vi "регистр на RSDC(фронтовой).vi"(2 "C":bool, 3 "S":bool, 4 "R":bool, 5 "d":T3) -> (0 "not q":T1, 1 "q":T2)   [LabVIEW 2012]
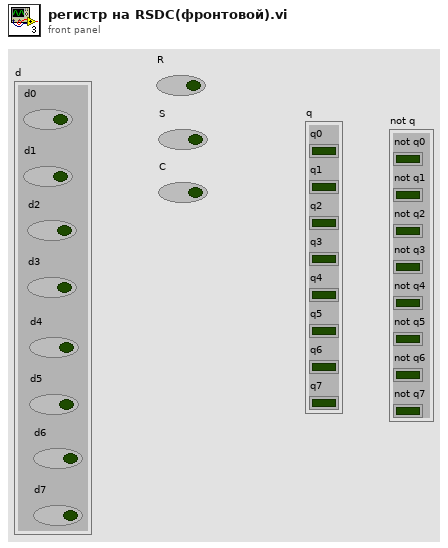
[diagram p1: front panel]
types:
  T1 = cluster{"not q0":bool, "not q1":bool, "not q2":bool, "not q3":bool, "not q4":bool, "not q5":bool, "not q6":bool, "not q7":bool}
  T2 = cluster{"q0":bool, "q1":bool, "q2":bool, "q3":bool, "q4":bool, "q5":bool, "q6":bool, "q7":bool}
  T3 = cluster{"d0":bool, "d1":bool, "d2":bool, "d3":bool, "d4":bool, "d5":bool, "d6":bool, "d7":bool}
  T4 = cluster{"Q":bool, "Q":bool, "Q":bool, "Q":bool, "Q":bool, "Q":bool, "Q":bool, "Q":bool}
  T5 = cluster{"not Q":bool, "not Q":bool, "not Q":bool, "not Q":bool, "not Q":bool, "not Q":bool, "not Q":bool, "not Q":bool}
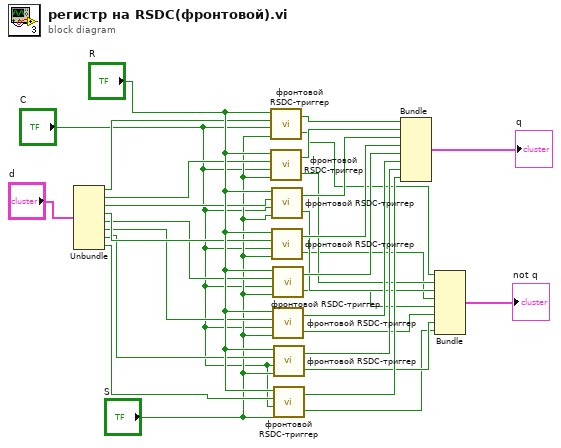
[diagram p0: block diagram]
diagram:
  n1 = Unbundle("d") -> ("d0"=w28:bool, "d1"=w27:bool, "d2"=w26:bool, "d3"=w25:bool, "d4"=w24:bool, "d5"=w23:bool, "d6"=w22:bool, "d7"=w21:bool)
  n2 = call "фронтовой RSDC-триггер.vi"("S"="S", "C"="C", "D"=w28, "R"="R") -> ("not Q"=w9:bool, "Q"=w18:bool)
  n3 = call "фронтовой RSDC-триггер.vi"("S"="S", "C"="C", "D"=w27, "R"="R") -> ("not Q"=w8:bool, "Q"=w17:bool)
  n4 = call "фронтовой RSDC-триггер.vi"("S"="S", "C"="C", "D"=w26, "R"="R") -> ("not Q"=w7:bool, "Q"=w16:bool)
  n5 = call "фронтовой RSDC-триггер.vi"("S"="S", "C"="C", "D"=w25, "R"="R") -> ("not Q"=w6:bool, "Q"=w15:bool)
  n6 = call "фронтовой RSDC-триггер.vi"("S"="S", "C"="C", "D"=w24, "R"="R") -> ("not Q"=w5:bool, "Q"=w14:bool)
  n7 = call "фронтовой RSDC-триггер.vi"("S"="S", "C"="C", "D"=w23, "R"="R") -> ("not Q"=w4:bool, "Q"=w13:bool)
  n8 = call "фронтовой RSDC-триггер.vi"("S"="S", "C"="C", "D"=w22, "R"="R") -> ("not Q"=w3:bool, "Q"=w12:bool)
  n9 = call "фронтовой RSDC-триггер.vi"("S"="S", "C"="C", "D"=w21, "R"="R") -> ("not Q"=w2:bool, "Q"=w11:bool)
  n10 = Bundle("Q"=w18, "Q"=w17, "Q"=w16, "Q"=w15, "Q"=w14, "Q"=w13, "Q"=w12, "Q"=w11) -> (→"q":T4)  [unwired: 1 in]
  n11 = Bundle("not Q"=w9, "not Q"=w8, "not Q"=w7, "not Q"=w6, "not Q"=w5, "not Q"=w4, "not Q"=w3, "not Q"=w2) -> (→"not q":T5)  [unwired: 1 in]
